vi "thermometer with average values.vi"() -> ()   [LabVIEW 2019]
panel:
  out "Waveform Chart":dbl(graph)
  in  "stop":bool
  out "Average of the last three temperatures":dbl
  in  "Temp Scale":bool
  # "deg C"
  # "deg F"
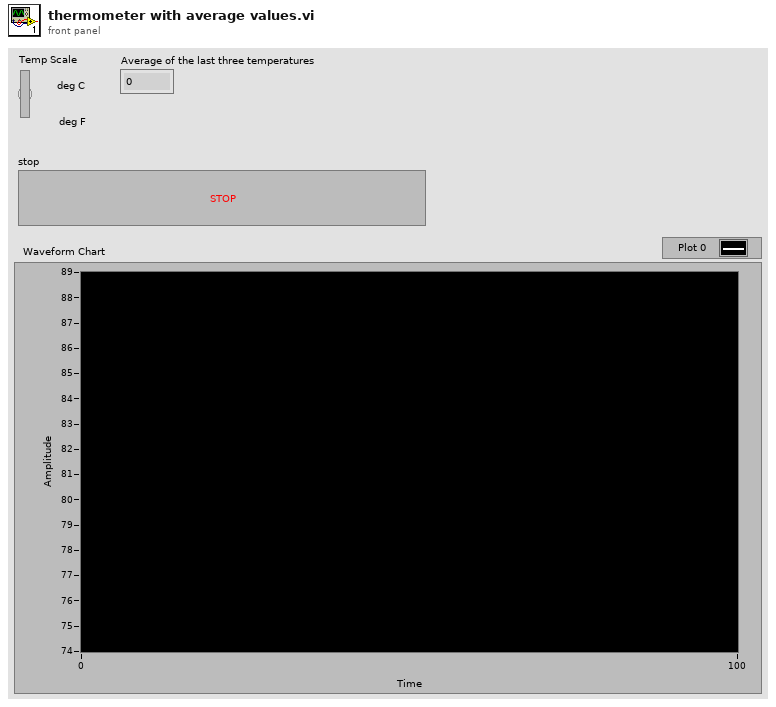
[diagram p1: front panel]
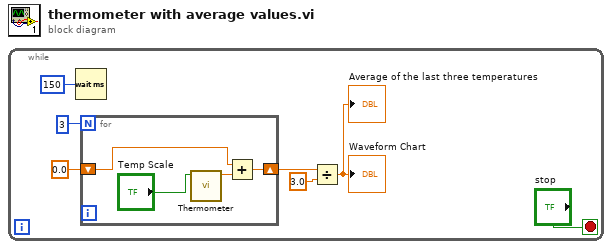
[diagram p0: block diagram]
diagram:
  n1 = while {
    stop <- "stop" stop-if-true
    n2 = Wait (ms)(milliseconds to wait=u32 150) -> ()  [unwired: 1 out]
    n3 = for {
      N: 3 -> [_]
      shift-right: [w10] -> w6
      shift-left: 0.0 -> [w8]
      n4 = call "Thermometer.vi"("Temp Scale"="Temp Scale") -> ("Temperature"=w9:dbl)  [unwired: 10 in]
      n5 = Add(x=w8, y=w9) -> (x+y=w10:dbl)
    }
    n6 = Divide(x=w6, y=3.0) -> (x/y=→"Average of the last three temperatures" →"Waveform Chart":dbl)
  }
